vi "CRYMake Operator ID.vi"(11 "sOperator Type":string) -> (0 "scope-fft mode":u32, 1 "VI nID":i32, 2 "Title ID":i32, 3 "Window Name":string)   [LabVIEW 2013]
uses:
  SubVI/CRYMisc vis settings global.vi
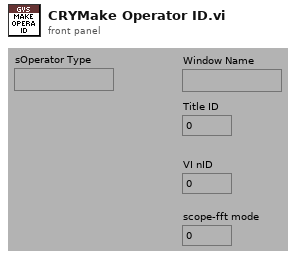
[diagram p1: front panel]
types:
  T1 = cluster{"VI Ref":refnum<vi>[], "VI nID":i32[], "Title nID":i32[]}
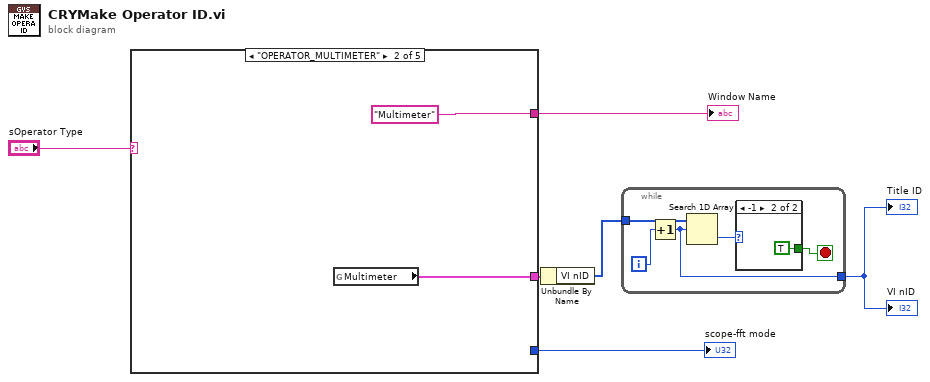
[diagram p0: block diagram]
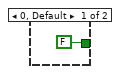
[diagram p2: hidden frame]
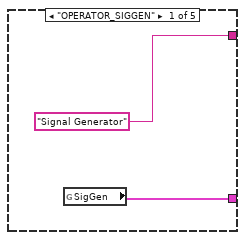
[diagram p3: hidden frame]
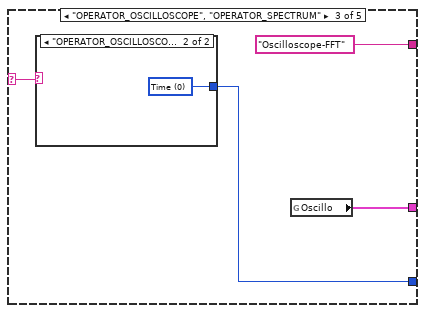
[diagram p4: hidden frame]
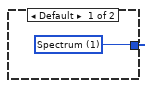
[diagram p5: hidden frame]
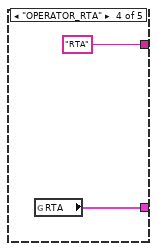
[diagram p6: hidden frame]
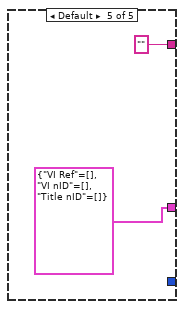
[diagram p7: hidden frame]
diagram:
  n1 = case shown="\"OPERATOR_MULTIMETER\"" "sOperator Type" {
    selector: "sOperator Type" -> [_ _ w13 _ _]
    tunnel: [w8 w10 w14 w18 T1 {"VI Ref"=[], "VI nID"=[], "Title nID"=[]} ("RTA")] -> w6
    tunnel: ["Signal Generator" ("sAction") "Multimeter" ("sAction") "Oscilloscope-FFT" ("sAction") "RTA" ("sAction") "" ("sAction")] -> w4
    tunnel: [_ _ w11 _ _] -> w3
    frame "OPERATOR_SIGGEN" {
      n2 = global read "CRYMisc vis settings global.vi" "SigGen"() -> (w8:T1)
    }
    frame "OPERATOR_MULTIMETER" {
      n3 = global read "CRYMisc vis settings global.vi" "Multimeter"() -> (w10:T1)
    }
    frame "OPERATOR_OSCILLOSCOPE", "OPERATOR_SPECTRUM" {
      n4 = case shown="\"OPERATOR_OSCILLOSCOPE\"" w13 {
        tunnel: [w15 w16] -> w11
        frame Default {
          w15 = u32 1 items=["Time", "Spectrum"] ("scope-fft mode")
        }
        frame "OPERATOR_OSCILLOSCOPE" {
          w16 = u32 0 items=["Time", "Spectrum"] ("scope-fft mode")
        }
      }
      n5 = global read "CRYMisc vis settings global.vi" "Oscillo"() -> (w14:T1)
    }
    frame "OPERATOR_RTA" {
      n6 = global read "CRYMisc vis settings global.vi" "RTA"() -> (w18:T1)
    }
    frame Default {
    }
  }
  "Window Name" <- w4
  "scope-fft mode" <- w3
  n7 = Unbundle By Name(w6) -> ("VI nID"=w2:i32[])
  n8 = while {
    tunnel: w2 -> [w25]
    tunnel: [w21] -> w1
    i -> [w24]
    stop <- w22 stop-if-true
    n9 = Increment(x=w24) -> (x+1=w21:i32)
    n10 = Search 1D Array(1D array=w25, element=w21) -> (index of element=w23:i32)  [unwired: 1 in]
    n11 = case shown="-1" w23 {
      tunnel: [FALSE TRUE] -> w22
      frame 0, Default {
      }
      frame -1 {
      }
    }
  }
  "Title ID" <- w1
  "VI nID" <- w1
